vi "Open.vi"(0 "SerialPortRef":T2, 5 "UpdateRate (100Hz)":u8=100, 9 "Nav6Mode (YPR)":T3, 11 "error in (no error)":errorcluster) -> (3 "Output Rate":u32, 4 "Nav6DevRef":T1, 6 "CalibrationState":T4, 8 "Gyroscope Full Scale Range":u32, 10 "Accelerometer Full Scale Range":u32, 14 "Open Succesfull":bool, 15 "error out":errorcluster)   [LabVIEW 2013, in "Nav6.lvlib"]
uses:
  Nav6.lvlib
  <vilib>/Rock Robotics/WPI/SerialPort/WPI_SerialPortRef.ctl
  Nav6Mode.ctl
  CalibrationState.ctl
  Nav6DevRef.ctl
  <vilib>/Utility/error.llb/DialogType.ctl
  <vilib>/Instr/_visa.llb/VISA Configure Serial Port (Instr).vi
  StopGlobal.vi
panel:
  out "Calibrated Yaw Offset":dbl
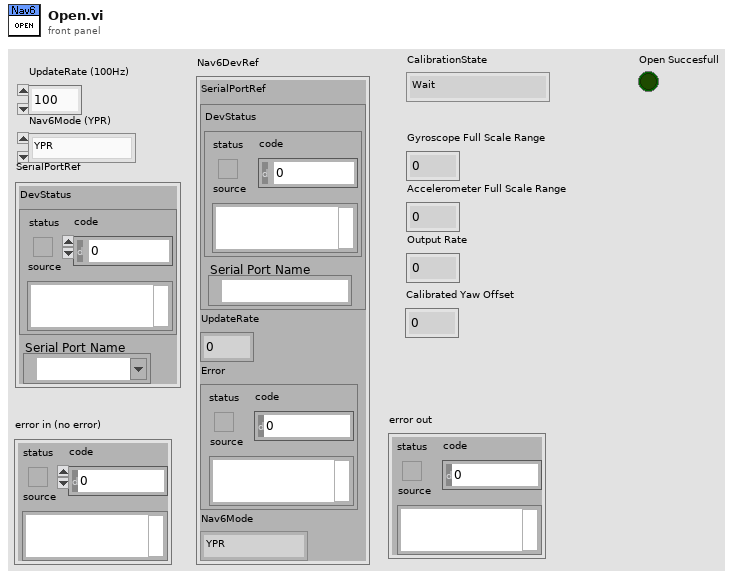
[diagram p1: front panel]
types:
  T1 = typedef "Nav6.lvlib/Nav6DevRef.ctl" = cluster{"SerialPortRef":T2, "UpdateRate":u8, "Error":errorcluster, "Nav6Mode":T3}
  T2 = typedef "WPI_SerialPortRef.ctl" = cluster{"DevStatus":errorcluster, "Serial Port Name":refnum<visa-resource-name>}
  T3 = typedef "Nav6.lvlib/Nav6Mode.ctl" = enum16{"YPR", "Gyro", "Quaternion"}
  T4 = typedef "Nav6.lvlib/CalibrationState.ctl" = enum16{"Wait", "Accumulate", "Complete"}
  T5 = typedef "DialogType.ctl" = u16
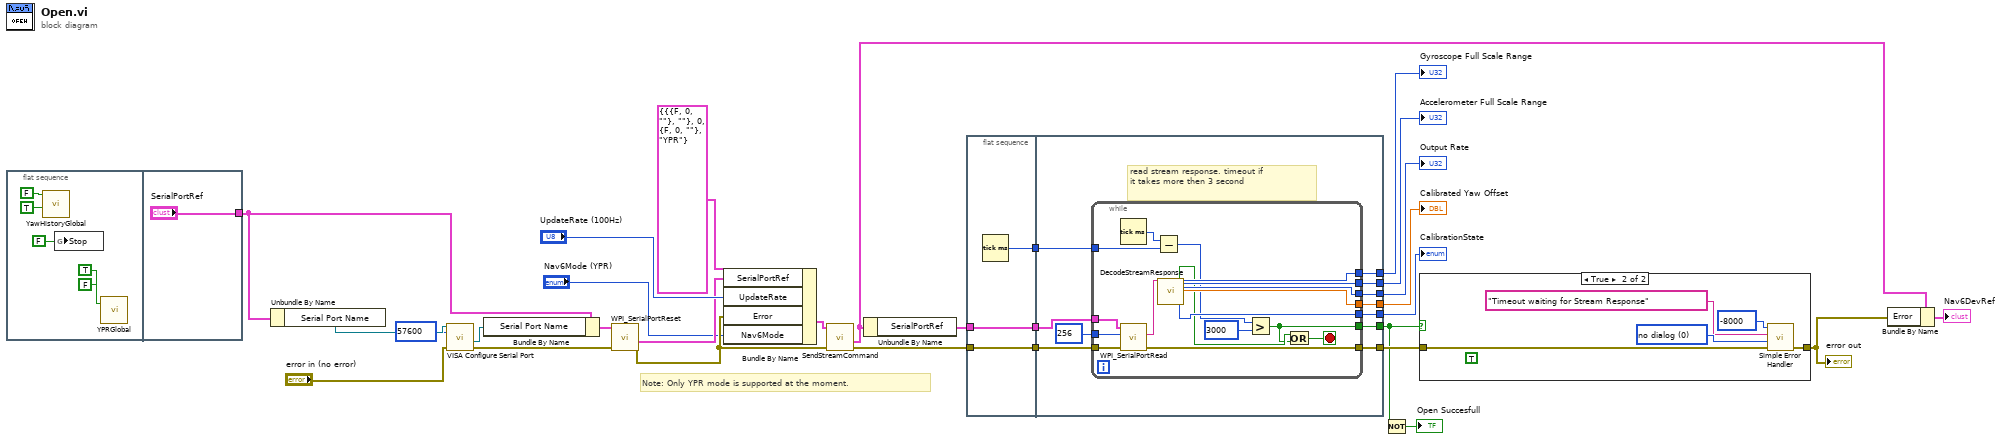
[diagram p0: block diagram]
diagram:
  # "Note: Only YPR mode is supported at the moment."
  n1 = flat-sequence {
    tunnel: ["SerialPortRef"] -> w8
    frame #0 {
      n2 = call "YawHistoryGlobal.vi"("Initialize"=TRUE, "Update"=FALSE) -> ()  [unwired: 9 in, 1 out]
      n3 = global write "StopGlobal.vi" "Stop"(FALSE ("Stop")) -> ()
      n4 = call "YPRGlobal.vi"("Update"=FALSE, "Initialize"=TRUE) -> ()  [unwired: 19 in, 7 out]
    }
    frame #1 {
    }
  }
  n5 = Unbundle By Name(w8) -> ("Serial Port Name"=w24:refnum<visa-resource-name>)
  n6 = call-poly "VISA Configure Serial Port"("VISA resource name"=w24, "baud rate (9600)"=u32 57600, "error in (no error)"="error in (no error)") -> ("VISA resource name out"=w22:refnum<visa-resource-name>, "error out"=w19:errorcluster)  [unwired: 11 in]
  n7 = Bundle By Name(cluster=w8, "Serial Port Name"=w22) -> (w21:T2)
  n8 = call <vilib>:"WPI_SerialPortReset.vi"("error in (no error)"=w19, "SerialPortRef"=w21) -> ("error out"=w26:errorcluster, "SerialPortRef"=w25:T2)  [unwired: 8 in]
  n9 = Bundle By Name(cluster=T1 {"SerialPortRef"={"DevStatus"={"status"=FALSE, "code"=0, "source"=""}, "Serial Port Name"=""}, "UpdateRate"=0, "Error"={"status"=FALSE, "code"=0, "source"=""}, "Nav6Mode"=enum."YPR"} ("Nav6DevRef"), "SerialPortRef"=w25, "UpdateRate"="UpdateRate (100Hz)", "Error"=w26, "Nav6Mode"="Nav6Mode (YPR)") -> (w28:T1)
  n10 = call "SendStreamCommand.vi"("error in (no error)"=w26, "Nav6DevRef"=w28) -> ("error out"=w12:errorcluster, "Nav6DevRef"=w5:T1)  [unwired: 8 in]
  n11 = Unbundle By Name(w5) -> ("SerialPortRef"=w13:T2)
  n12 = flat-sequence {
    tunnel: w12 -> [w37]
    tunnel: w13 -> [w38]
    tunnel: [w38] -> w4
    tunnel: [w37] -> w3
    tunnel: [w36] -> w2
    tunnel: [w49] -> w18
    tunnel: [w48] -> w17
    tunnel: [w47] -> w16
    tunnel: [w46] -> w15
    tunnel: [w42] -> w11
    tunnel: [w41] -> w10
    tunnel: [w40] -> w9
    tunnel: w4 -> [w45]
    tunnel: w3 -> [w44]
    tunnel: w2 -> [w39]
    frame #0 {
      n13 = Tick Count (ms)() -> (millisecond timer value=w36:u32)
    }
    frame #1 {
      # "read stream response. timeout if\nit takes more then 3 second"
      n14 = while {
        tunnel: [w66] -> w49
        tunnel: [w65] -> w48
        tunnel: [w64] -> w47
        tunnel: [w63] -> w46
        tunnel: [w62] -> w41
        tunnel: w45 -> [w61]
        tunnel: w44 -> [w60]
        tunnel: u32 256 ("Num Bytes to Read") -> [w58]
        tunnel: [w57] -> w42
        tunnel: w39 -> [w51]
        tunnel: [w50] -> w40
        stop <- w53 stop-if-true
        n15 = Tick Count (ms)() -> (millisecond timer value=w52:u32)
        n16 = call <vilib>:"WPI_SerialPortRead.vi"("error in (no error)"=w60, "Num Bytes to Read"=w58, "SerialPortRef"=w61) -> ("error out"=w62:errorcluster, "Buffer"=w59:string)  [unwired: 6 in, 1 out]
        n17 = Subtract(x=w52, y=w51) -> (x-y=w56:u32)
        n18 = call "DecodeStreamResponse.vi"("Buffer"=w59) -> ("ChecksumVerified"=w54:bool, "Flags"=w57:u32, "Gyroscope Full Scale Range"=w66:u32, "Accelerometer Full Scale Range"=w65:u32, "Output Rate"=w64:u32, "Calibrated Yaw Offset"=w63:dbl)  [unwired: 17 in, 4 out]
        n19 = Greater?(x=w56, y=u32 3000) -> (0:w50:bool)
        n20 = Or(x=w54, y=w50) -> (x .or. y?=w53:bool)
      }
    }
  }
  n21 = Not(x=w9) -> (.not. x?=→"Open Succesfull":bool)
  n22 = case shown="True" w9 {
    tunnel: w10 -> [w67 w69]
    tunnel: [w67 w68] -> w6
    frame False {
    }
    frame True {
      (unwired) TRUE ("Update")
      w72 = T5 0 items=["no dialog", "OK message", "continue or stop message", "OK message + warnings", "continue/stop + warnings"] ("type of dialog (OK msg:1)")
      n23 = call <vilib>:"Simple Error Handler.vi"("error code (no error:0)"=-8000, "error source (\" \")"="Timeout waiting for Stream Response" ("error source (\" \")"), "type of dialog (OK msg:1)"=w72, "error in (no error)"=w69) -> ("error out"=w68:errorcluster)  [unwired: 1 in, 4 out]
    }
  }
  "error out" <- w6
  n24 = Bundle By Name(cluster=w5, "Error"=w6) -> (→"Nav6DevRef":T1)
  "Calibrated Yaw Offset" <- w15
  "Output Rate" <- w16
  "Accelerometer Full Scale Range" <- w17
  "Gyroscope Full Scale Range" <- w18
  "CalibrationState" <- w11
